vi "Cal Tank Data.vi"(0 "Cal Coefficients":dbl[][](array[numeric])=[[0.0, 1.0, 0.0], [0.0, 1.0, 0.0], [0.0, 1.0, 0.0], [0.0, 1.0, 0.0], [0.0, 1.0, 0.0], [0.0, 1.0, 0.0], [0.0, 1.0, 0.0], [0.0, 1.0, 0.0], [0.0, 1.0, 0.0], [0.0, 1.0, 0.0], [0.0, 1.0, 0.0], [0.0, 1.0, 0.0], [0.0, 1.0, 0.0], [0.0, 1.0, 0.0], [0.0, 1.0, 0.0], [0.0, 1.0, 0.0], [0.0, 1.0, 0.0], [0.0, 1.0, 0.0], [0.0, 1.0, 0.0], [0.0, 1.0, 0.0], [0.0, 1.0, 0.0], [0.0, 1.0, 0.0], [0.0, 1.0, 0.0], [0.0, 1.0, 0.0], [0.0, 1.0, 0.0], [0.0, 1.0, 0.0], [0.0, 1.0, 0.0], [0.0, 1.0, 0.0], [0.0, 1.0, 0.0], [0.0, 1.0, 0.0], [0.0, 1.0, 0.0], [0.0, 1.0, 0.0], [0.0, 1.0, 0.0], [0.0, 1.0, 0.0], [0.0, 1.0, 0.0], [0.0, 1.0, 0.0], [0.0, 1.0, 0.0], [0.0, 1.0, 0.0], [0.0, 1.0, 0.0], [0.0, 1.0, 0.0], [0.0, 1.0, 0.0], [0.0, 1.0, 0.0], [0.0, 1.0, 0.0], [0.0, 1.0, 0.0]], 11 "Raw Tank Data":dbl[](array[numeric])) -> (4 "Data Out":dbl[](array[numeric]))   [LabVIEW 2019]
uses:
  <vilib>/ptbypt/NI_PtbyPt.lvlib
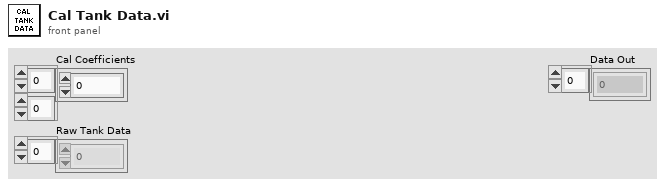
[diagram p1: front panel]
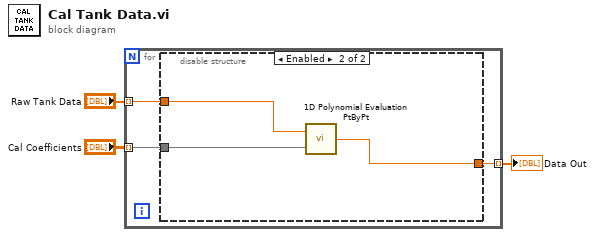
[diagram p0: block diagram]
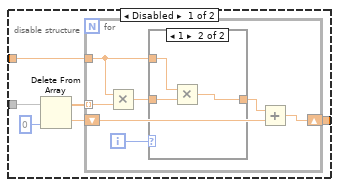
[diagram p2: hidden frame]
diagram:
  n1 = for {
    tunnel: "Raw Tank Data" -> [w6] mode=indexing
    tunnel: "Cal Coefficients" -> [w5] mode=indexing
    tunnel: [w4] -> w1 mode=indexing
    n2 = disable-structure shown="Enabled" {
      disable-tunnel: w6 -> [w12 w25]
      disable-tunnel: w5 -> [w11 w26]
      disable-tunnel: [w7 w24] -> w4
      frame Disabled {
        n3 = Delete From Array(array=w11, index=0) -> (deleted portion=w9:dbl, array with subset deleted=w8:dbl[])  [unwired: 1 in]
        n4 = for {
          tunnel: w12 -> [w18]
          shift-right: [w13] -> w7
          shift-left: w9 -> [w15]
          tunnel: w8 -> [w17] mode=indexing
          i -> [w19]
          n5 = Multiply(x=w18, y=w17) -> (x*y=w16:dbl)
          n6 = case shown="1" w19 {
            tunnel: w18 -> [_ w22]
            tunnel: w16 -> [w20 w23]
            tunnel: [w20 w21] -> w14
            frame 0, Default {
            }
            frame 1 {
              n7 = Multiply(x=w22, y=w23) -> (x*y=w21:dbl)
            }
          }
          n8 = Add(x=w14, y=w15) -> (x+y=w13:dbl)
        }
      }
      frame Enabled {
        n9 = call <vilib>:"1D Polynomial Evaluation PtByPt.vi"("Coefficients: a"=w26, "x"=w25) -> ("y"=w24:dbl)
      }
    }
  }
  "Data Out" <- w1
